vi "DAQ_sub_DI-DO_.vi"(8 "error in":errorcluster, 9 "All OFF":bool, 10 "ON/OFF":bool=TRUE, 11 "Channel":i32) -> (0 "error out":errorcluster, 3 "DigitalRead":bool)   [LabVIEW 2021]
uses:
  <vilib>/DAQmx/read.llb/DAQmx Read (Digital Bool 1Line 1Point).vi
  <vilib>/DAQmx/write.llb/DAQmx Write (Digital Bool 1Line 1Point).vi
  <vilib>/DAQmx/write.llb/DAQmx Write (Digital 1D Bool 1Chan 1Samp).vi
  <vilib>/DAQmx/create/channels.llb/DAQmx Create Channel (DI-Digital Input).vi
  <vilib>/DAQmx/miscellaneous.llb/DAQmx Fill In Error Info.vi
  <vilib>/DAQmx/create/channels.llb/DAQmx Create Channel (DO-Digital Output).vi
panel:
  in  "auto start 2":bool=TRUE
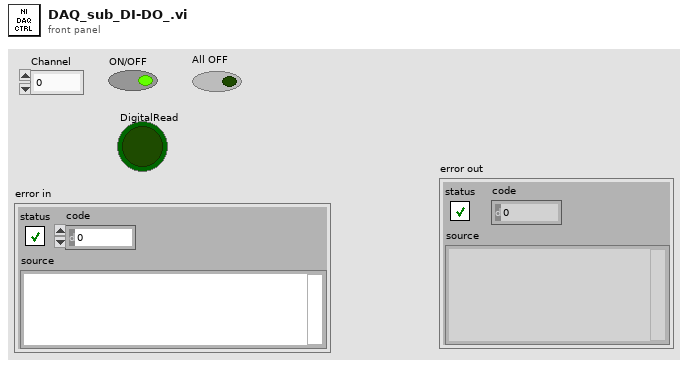
[diagram p1: front panel]
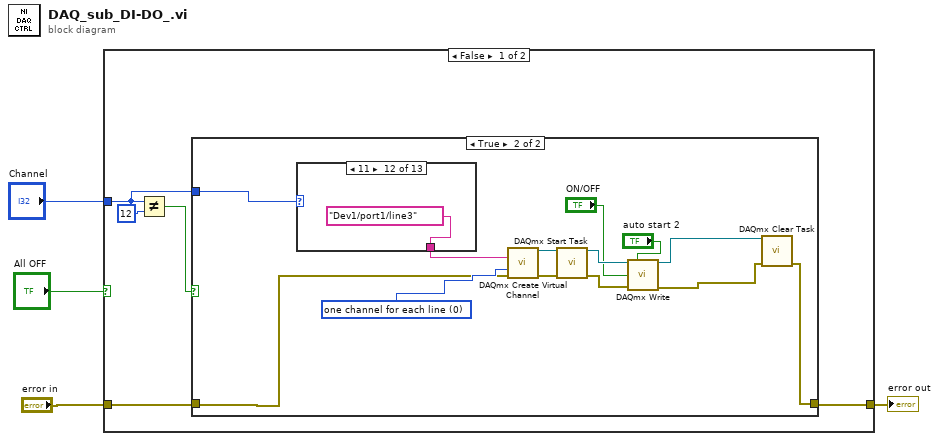
[diagram p0: block diagram]
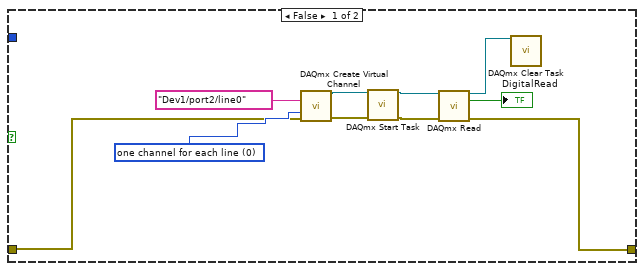
[diagram p2: hidden frame]
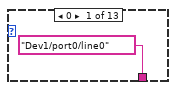
[diagram p3: hidden frame]
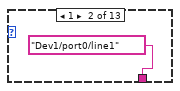
[diagram p4: hidden frame]
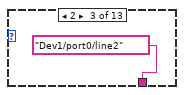
[diagram p5: hidden frame]
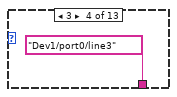
[diagram p6: hidden frame]
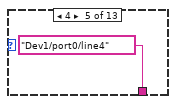
[diagram p7: hidden frame]
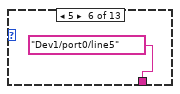
[diagram p8: hidden frame]
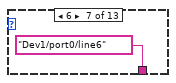
[diagram p9: hidden frame]
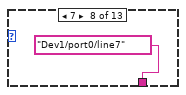
[diagram p10: hidden frame]
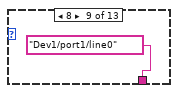
[diagram p11: hidden frame]
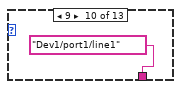
[diagram p12: hidden frame]
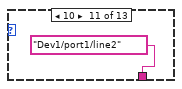
[diagram p13: hidden frame]
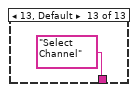
[diagram p14: hidden frame]
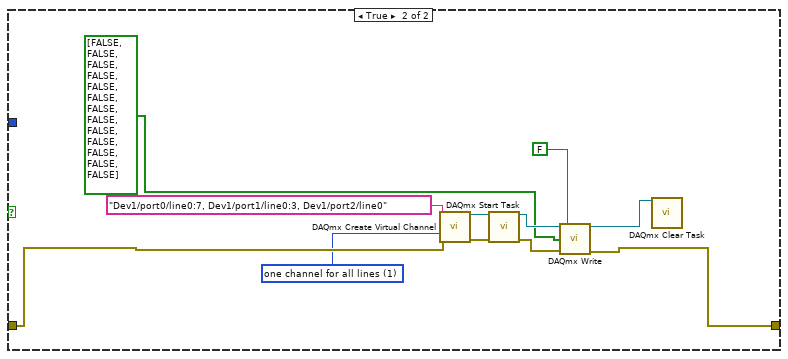
[diagram p15: hidden frame]
diagram:
  n1 = case shown="False" "All OFF" {
    tunnel: "Channel" -> [w6 _]
    tunnel: "error in" -> [w9 w56]
    tunnel: [w8 w55] -> w1
    frame False {
      n2 = Not Equal?(x=w6, y=12) -> (x != y?=w5:bool)
      n3 = case shown="True" w5 {
        tunnel: w9 -> [w18 w26]
        tunnel: [w12 w20] -> w8
        tunnel: w6 -> [_ w23]
        frame False {
          w19 = 0 items=["one channel for each line", "one channel for all lines"] ("line grouping")
          n4 = call-poly <vilib>:"DAQmx Create Virtual Channel.vi"("lines"=tag "Dev1/port2/line0", "line grouping"=w19, "error in"=w18) -> ("task out"=w16:refnum<k21>, "error out"=w15:errorcluster)  [unwired: 11 in]
          n5 = call <vilib>:"DAQmx Start Task.vi"("task/channels in"=w16, "error in"=w15) -> ("task out"=w14:refnum<k21>, "error out"=w13:errorcluster)  [unwired: 12 in]
          n6 = call-poly <vilib>:"DAQmx Read.vi"("task/channels in"=w14, "error in"=w13) -> ("task out"=w10:refnum<k21>, "data"=→"DigitalRead":bool, "error out"=w12:errorcluster)  [unwired: 11 in]
          n7 = call <vilib>:"DAQmx Clear Task.vi"("task in"=w10) -> ()  [unwired: 14 in, 1 out]
        }
        frame True {
          w30 = 0 items=["one channel for each line", "one channel for all lines"] ("line grouping")
          n8 = case shown="11" w23 {
            tunnel: [tag "Dev1/port0/line0" ("lines") tag "Dev1/port0/line1" ("lines 2") tag "Dev1/port0/line2" ("lines 2") tag "Dev1/port0/line3" ("lines 2") tag "Dev1/port0/line4" ("lines 2") tag "Dev1/port0/line5" ("lines 2") tag "Dev1/port0/line6" ("lines 2") tag "Dev1/port0/line7" ("lines 2") tag "Dev1/port1/line0" ("lines 2") tag "Dev1/port1/line1" ("lines 2") tag "Dev1/port1/line2" ("lines 2") tag "Dev1/port1/line3" ("lines 2") "Select Channel"] -> w27
            frame 0 {
            }
            frame 1 {
            }
            frame 2 {
            }
            frame 3 {
            }
            frame 4 {
            }
            frame 5 {
            }
            frame 6 {
            }
            frame 7 {
            }
            frame 8 {
            }
            frame 9 {
            }
            frame 10 {
            }
            frame 11 {
            }
            frame 13, Default {
            }
          }
          n9 = call-poly <vilib>:"DAQmx Create Virtual Channel.vi"("lines"=w27, "line grouping"=w30, "error in"=w26) -> ("task out"=w29:refnum<k21>, "error out"=w25:errorcluster)  [unwired: 11 in]
          n10 = call <vilib>:"DAQmx Start Task.vi"("task/channels in"=w29, "error in"=w25) -> ("task out"=w31:refnum<k21>, "error out"=w24:errorcluster)  [unwired: 12 in]
          n11 = call-poly <vilib>:"DAQmx Write.vi"("task/channels in"=w31, "auto start"="auto start 2", "data"="ON/OFF", "error in"=w24) -> ("task out"=w22:refnum<k21>, "error out"=w21:errorcluster)  [unwired: 9 in, 1 out]
          n12 = call <vilib>:"DAQmx Clear Task.vi"("task in"=w22, "error in"=w21) -> ("error out"=w20:errorcluster)  [unwired: 13 in]
        }
      }
    }
    frame True {
      w53 = 1 items=["one channel for each line", "one channel for all lines"] ("line grouping")
      n13 = call-poly <vilib>:"DAQmx Create Virtual Channel.vi"("lines"=tag "Dev1/port0/line0:7, Dev1/port1/line0:3, Dev1/port2/line0", "line grouping"=w53, "error in"=w56) -> ("task out"=w52:refnum<k21>, "error out"=w51:errorcluster)  [unwired: 11 in]
      n14 = call <vilib>:"DAQmx Start Task.vi"("task/channels in"=w52, "error in"=w51) -> ("task out"=w54:refnum<k21>, "error out"=w50:errorcluster)  [unwired: 12 in]
      n15 = call-poly <vilib>:"DAQmx Write.vi"("task/channels in"=w54, "auto start"=FALSE, "data"=bool[] [FALSE, FALSE, FALSE, FALSE, FALSE, FALSE, FALSE, FALSE, FALSE, FALSE, FALSE, FALSE, FALSE], "error in"=w50) -> ("task out"=w46:refnum<k21>, "error out"=w55:errorcluster)  [unwired: 9 in, 1 out]
      n16 = call <vilib>:"DAQmx Clear Task.vi"("task in"=w46) -> ()  [unwired: 14 in, 1 out]
    }
  }
  "error out" <- w1
